vi "UpdatePlugins.vi"(0 "Current Paths":path[](array[path]), 1 "rngInst":refnum<vi>, 2 "Priority":u8=2, 3 "Severity (Critical)":string="Critical", 5 "Instrument Modules":T1=[{"PluginSelection"=1, "ConfigDialog"=FALSE}, {"PluginSelection"=11, "ConfigDialog"=FALSE}] {"PluginSelection" items=["C37.118 PMU", "C37.118 Sim", "Base PMU", "none", "SiemensDEM0", "AcPwrBase", "Chroma0", "Chroma1", "Chroma2", "NHRDC0", "NHRRGS0", "PPS0"]}, 11 "Error In Array":errorcluster[](array[cluster])) -> (4 "Current Paths":string[](array[string])=["..\\UserFiles\\Plugins\\AcPwr", "..\\UserFiles\\Plugins\\Sensor"], 14 "PluginTypes":string[](array[string]), 15 "Error Out Array":errorcluster[](array[cluster]))   [LabVIEW 2018]
doc: "This VI allows the user to update which Plugins can be selected at the application layer by modifing the location(s) of the INI file(s)."
uses:
  Framework/InstrumentModulesControl.ctl
  <userlib>/NIST/NISTErrorLib/NISTErrorLib.lvlib
panel:
  in  "Save Button":bool
  in  "Update Plugins":bool
  in  "Instrument Modules":T1=[{"PluginSelection"=4, "ConfigDialog"=FALSE}] {"PluginSelection" items=["C37.118 PMU", "C37.118 Sim", "Base PMU", "none", "SiemensDEM0", "AcPwrBase", "Chroma0", "Chroma1", "Chroma2", "NHRDC0", "NHRRGS0", "PPS0"]}
  in  "Cancel  Button":bool
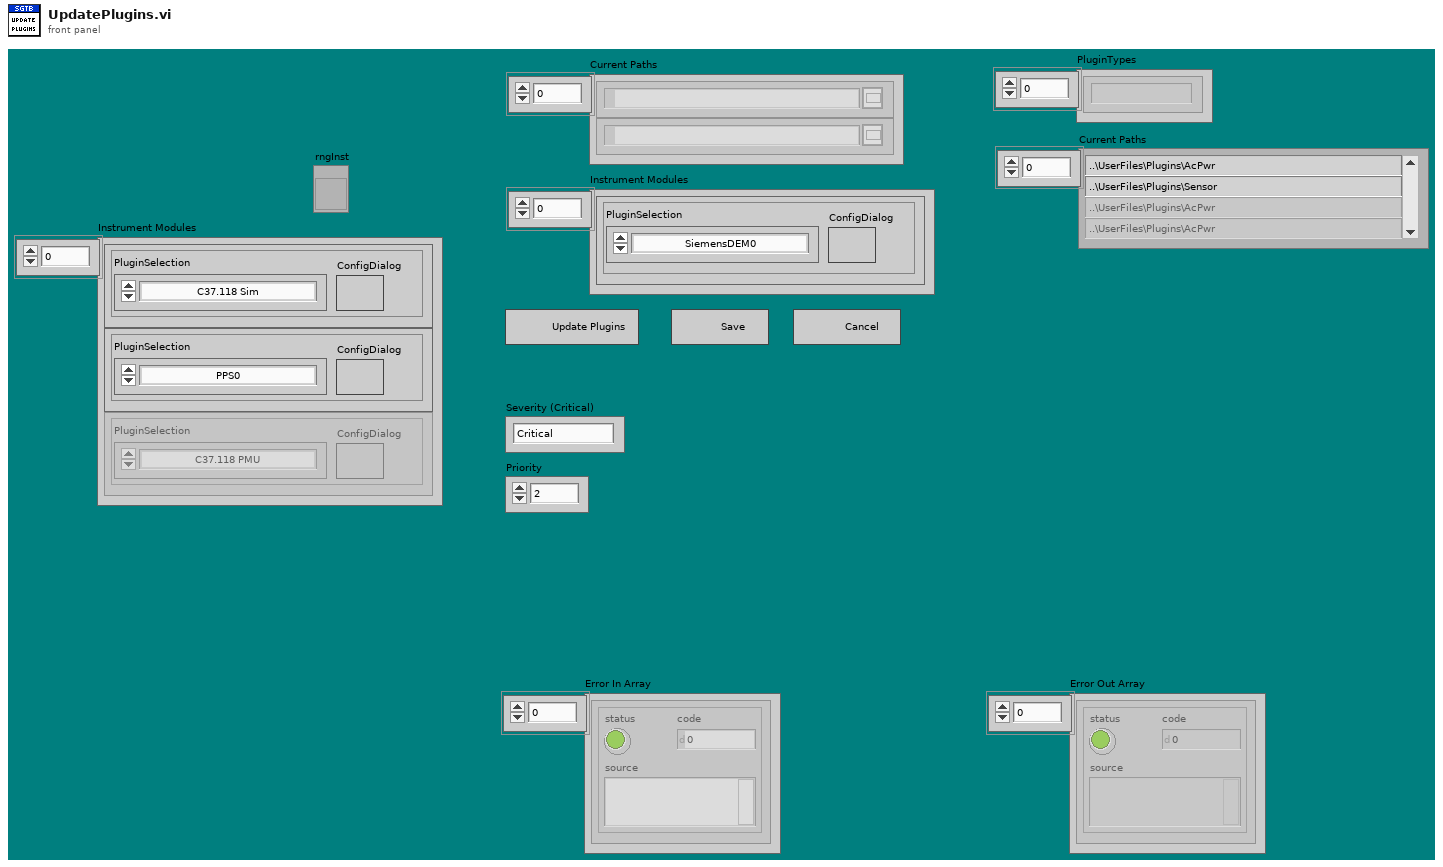
[diagram p1: front panel]
types:
  T1 = typedef "InstrumentModulesControl.ctl" = cluster{"PluginSelection":u16, "ConfigDialog":bool}[]
  T2 = enum32{"Invalid", "Standard", "Closed", "Hidden", "Minimized", "Maximized"}
  T3 = enum32{"Invalid", "Default", "Floating", "Floating/Auto-Hide", "Modal"}
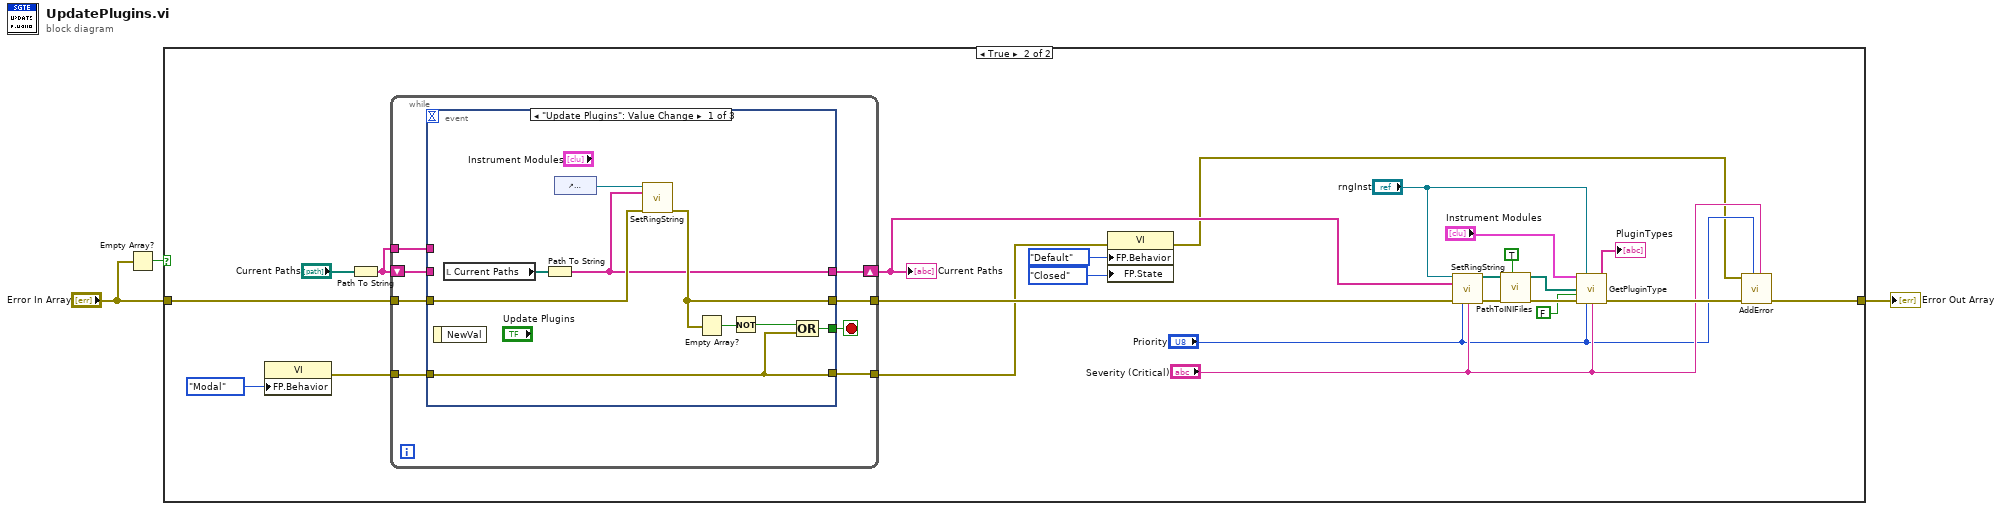
[diagram p0: block diagram]
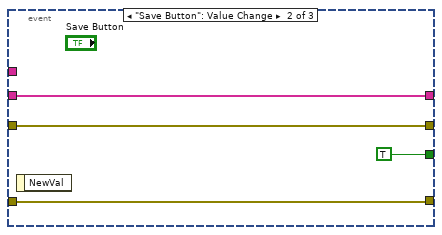
[diagram p3: hidden frame]
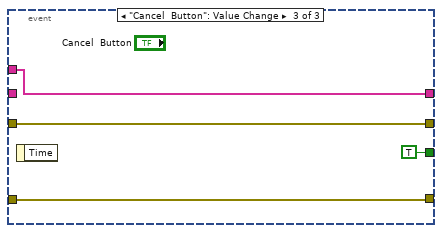
[diagram p4: hidden frame]
diagram:
  n1 = Empty Array?(array="Error In Array") -> (empty?=w2:bool)
  n2 = case shown="True" w2 {
    tunnel: "Error In Array" -> [w4 w27]
    tunnel: [w4 w8] -> w1
    frame False {
    }
    frame True {
      n3 = property class="VI"("FP.Behavior"=T3."Modal" ("Front Panel Window:Behavior")) -> (error out=w25:errorcluster)  [unwired: 2 in, 1 out]
      n4 = Path To String(path="Current Paths") -> (string=w10:string[])
      n5 = while {
        tunnel: w27 -> [w35]
        tunnel: [w33] -> w22
        tunnel: w25 -> [w32]
        tunnel: [w29] -> w21
        shift-right: [w30] -> w13
        shift-left: w10 -> [w31]
        tunnel: w10 -> [w28]
        stop <- w34 stop-if-true
        n6 = event shown="[0] \"Update Plugins\": Value Change" {
          selector: _ -> [_ _ _]
          dyn-events: _ -> [_ _ _]
          timeout: _ -> [_ _ _]
          tunnel: w35 -> [w44 w47 w51]
          tunnel: [w41 TRUE TRUE] -> w34
          tunnel: [w40 w47 w51] -> w33
          tunnel: w32 -> [w38 w45 w50]
          tunnel: w31 -> [_ w46 _]
          tunnel: [w36 w46 w52] -> w30
          tunnel: [w38 w45 w50] -> w29
          tunnel: w28 -> [_ _ w52]
          event "Update Plugins": Value Change {
            n7 = event-data() -> ()  [unwired: 1 in, 1 out]
            n8 = local read "Current Paths"() -> (w37:path[])
            n9 = Path To String(path=w37) -> (string=w36:string[])
            n10 = control-ref of="PluginSelection"() -> (w39:refnum<vi>)
            n11 = call "SetRingString.vi"("Ring in"=w39, "RelativePathToINIFiles"=w36, "ErrorArray In"=w44) -> ("ErrorArray Out out"=w40:errorcluster[])  [unwired: 11 in, 1 out]
            n12 = Empty Array?(array=w40) -> (empty?=w43:bool)
            n13 = Not(x=w43) -> (.not. x?=w42:bool)
            n14 = Compound Arithmetic op=OR(w42, w38) -> (w41:bool)
          }
          event "Save Button": Value Change {
            n15 = event-data() -> ()  [unwired: 1 in, 1 out]
          }
          event "Cancel  Button": Value Change {
            n16 = event-data() -> ()  [unwired: 1 in, 1 out]
          }
        }
      }
      "Current Paths" <- w13
      n17 = property class="VI"(error in=w21, "FP.Behavior"=T3."Default" ("Front Panel Window:Behavior"), "FP.State"=T2."Closed" ("Front Panel Window:State")) -> (error out=w5:errorcluster)  [unwired: 1 in, 1 out]
      n18 = call "SetRingString.vi"("Ring in"="rngInst", "RelativePathToINIFiles"=w13, "ErrorArray In"=w22, "Priority(2)"="Priority", "Severity(Critical)"="Severity (Critical)") -> ("IniFilePaths"=w17:path[], "ErrorArray Out out"=w16:errorcluster[])  [unwired: 9 in]
      n19 = call "PathToINIFiles.vi"("Boolean"=TRUE, "IniFilePaths In"=w17) -> ("IniFilePaths Out"=w18:path[])  [unwired: 9 in]
      n20 = call "GetPluginType.vi"("Instrument Modules In New"="Instrument Modules", "reference"="rngInst", "INIFilePaths"=w18, "Compare? (F)"=FALSE, "ErrorArray In"=w16, "Priority (2)"="Priority", "Severity (Critical)"="Severity (Critical)") -> ("PluginTypes"=→"PluginTypes":string[], "ErrorArray Out"=w9:errorcluster[])  [unwired: 4 in, 3 out]
      n21 = call <userlib>:"AddError.vi"("Severity"="Severity (Critical)", "Priority"="Priority", "ErrorArray In"=w9, "error in (no error)"=w5) -> ("ErrorArray Out"=w8:errorcluster[])  [unwired: 6 in, 1 out]
    }
  }
  "Error Out Array" <- w1
